vi "Add-to-log.vi"(8 "error in (no error)":errorcluster, 11 "Errors in":T1) -> (0 "error out":errorcluster, 3 "Errors out":T1)   [LabVIEW 2013, in "Error-handling.lvlib" / "Errors.lvclass"]
uses:
  Errors.lvclass
  Object-reference.ctl
  <vilib>/Utility/error.llb/DialogType.ctl
  Errors.lvclass/Errors.ctl
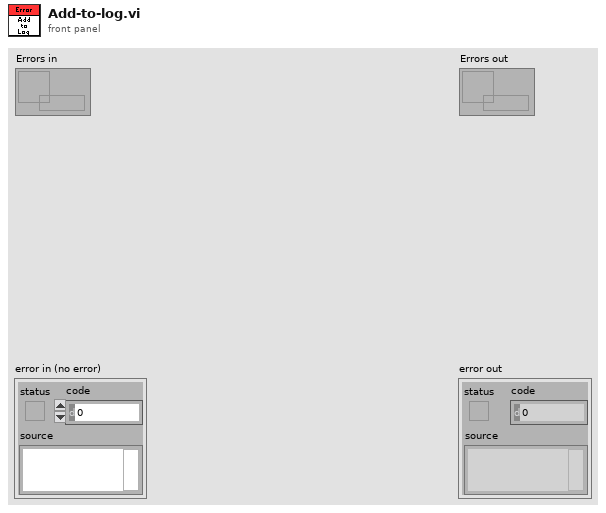
[diagram p1: front panel]
types:
  T1 = typedef "Error-handling.lvlib/Errors.lvclass/Object-reference.ctl" = refnum<data-value>
  T2 = typedef "DialogType.ctl" = u16
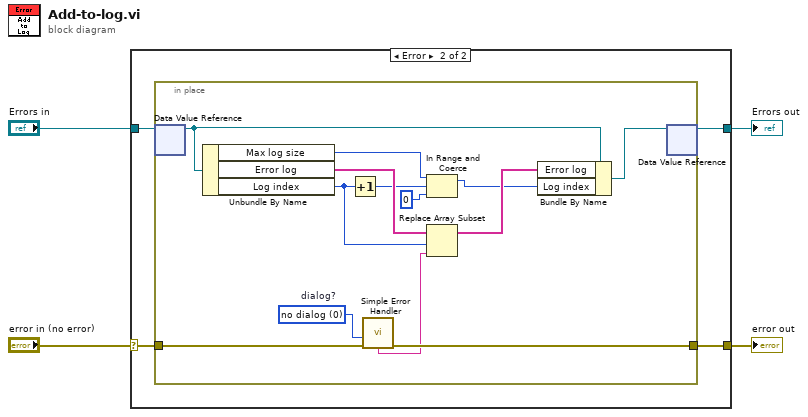
[diagram p0: block diagram]
diagram:
  n1 = case shown="Error" "error in (no error)" {
    selector: "error in (no error)" -> [w6 w8]
    tunnel: [w6 w7] -> w3
    tunnel: [w5 w9] -> w1
    tunnel: "Errors in" -> [w5 w10]
    frame No Error {
    }
    frame Error {
      n2 = in-place {
        in-place-border: w8 -> [w23]
        in-place-border: [w22] -> w7
        w21 = T2 0 items=["no dialog", "OK message", "continue or stop message", "OK message + warnings", "continue/stop + warnings"]  # dialog?
        n3 = in-place-dvr #1(w10) -> (w17:refnum<class "Errors.lvclass">)  [unwired: 1 out]
        n4 = Unbundle By Name(w17) -> ("Max log size"=w12:i32, "Error log"=w20:string[], "Log index"=w16:i32)
        n5 = Increment(x=w16) -> (x+1=w15:i32)
        n6 = call <vilib>:"Simple Error Handler.vi"("type of dialog (OK msg:1)"=w21, "error in (no error)"=w23) -> ("error out"=w22:errorcluster, "message"=w19:string)  [unwired: 3 in, 3 out]
        n7 = In Range and Coerce(upper limit=w12, x=w15, lower limit=0) -> (coerced(x)=w14:i32)  [unwired: 1 out]
        n8 = Replace Array Subset(array=w20, new element=w19, index=w16) -> (w18:string[])
        n9 = Bundle By Name(cluster=w17, "Error log"=w18, "Log index"=w14) -> (w13:refnum<class "Errors.lvclass">)
        n10 = in-place-dvr #1(w13) -> (w9:T1)  [unwired: 1 out]
      }
    }
  }
  "error out" <- w3
  "Errors out" <- w1
